vi "StellarNet MS Sw ini read I32.vi"(3 "Error State (In)":errorcluster, 4 "Section":string, 5 "configuration file path":path, 6 "Keys":string[](array[string])=["C1a", "C1b", "C1c", "C2d"]) -> (0 "Error State (Out)":errorcluster, 1 "Multi Elements":i32[](array[numeric]), 2 "Single Element":i32)   [LabVIEW 2023]
uses:
  <vilib>/Utility/config.llb/Read Key (I32).vi
  <vilib>/Utility/config.llb/NI_LVConfig.lvlib
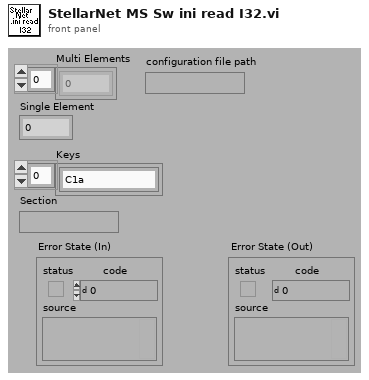
[diagram p1: front panel]
types:
  T1 = typedef "NI_LVConfig.lvlib/Config Data RefNum.ctl" = refnum<k1>
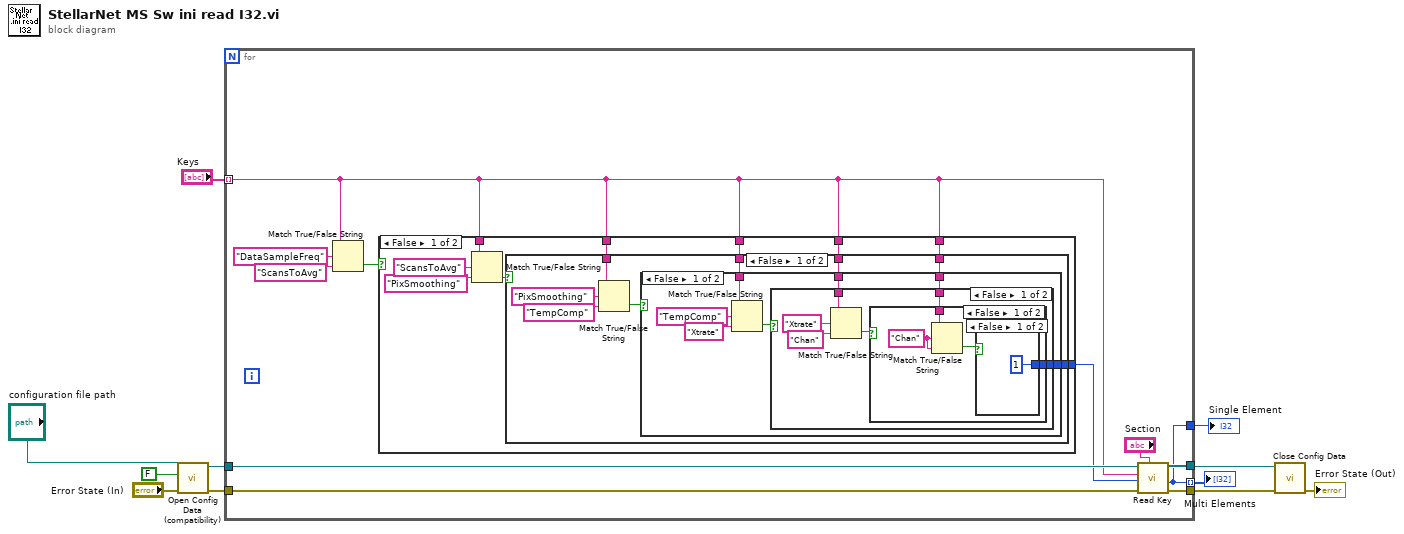
[diagram p0: block diagram]
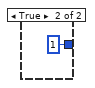
[diagram p2: hidden frame]
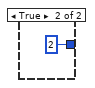
[diagram p3: hidden frame]
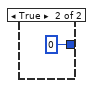
[diagram p4: hidden frame]
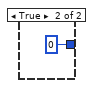
[diagram p5: hidden frame]
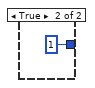
[diagram p6: hidden frame]
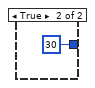
[diagram p7: hidden frame]
diagram:
  n1 = call <vilib>:"Open Config Data (compatibility).vi"("error in (no error)"="Error State (In)", "create file if necessary (T)"=FALSE ("create file if necessary? (T)"), "configuration file path"="configuration file path") -> ("error out"=w10:errorcluster, "refnum"=w9:T1)  [unwired: 6 in, 1 out]
  n2 = for {
    tunnel: w10 -> [w22]
    tunnel: w9 -> [w21]
    tunnel: "Keys" -> [w14] mode=indexing
    tunnel: [w18] -> w6 mode=indexing
    tunnel: [w20] -> w8
    tunnel: [w19] -> w7
    tunnel: [w18] -> w5
    n3 = Match True/False String(2:"ScansToAvg" ("regular expression"), 3:"DataSampleFreq" ("regular expression"), 4:w14) -> (0:w16:bool)  [unwired: 1 out]
    n4 = case shown="False" w16 {
      tunnel: w14 -> [w29 _]
      tunnel: w14 -> [w28 _]
      tunnel: w14 -> [w27 _]
      tunnel: w14 -> [w26 _]
      tunnel: w14 -> [w25 _]
      tunnel: [w24 30] -> w13
      frame False {
        n5 = Match True/False String(2:"PixSmoothing" ("regular expression"), 3:"ScansToAvg" ("regular expression"), 4:w29) -> (0:w30:bool)  [unwired: 1 out]
        n6 = case shown="False" w30 {
          tunnel: w28 -> [w38 _]
          tunnel: w27 -> [w36 _]
          tunnel: w26 -> [w35 _]
          tunnel: w25 -> [w34 _]
          tunnel: [w33 1] -> w24
          frame False {
            n7 = Match True/False String(2:"TempComp" ("regular expression"), 3:"PixSmoothing" ("regular expression"), 4:w38) -> (0:w37:bool)  [unwired: 1 out]
            n8 = case shown="False" w37 {
              tunnel: w36 -> [w45 _]
              tunnel: w35 -> [w44 _]
              tunnel: w34 -> [w42 _]
              tunnel: [w41 0] -> w33
              frame False {
                n9 = Match True/False String(2:"Xtrate" ("regular expression"), 3:"TempComp" ("regular expression"), 4:w45) -> (0:w43:bool)  [unwired: 1 out]
                n10 = case shown="False" w43 {
                  tunnel: w44 -> [w51 _]
                  tunnel: w42 -> [w49 _]
                  tunnel: [w48 0] -> w41
                  frame False {
                    n11 = Match True/False String(2:"Chan" ("regular expression"), 3:"Xtrate" ("regular expression"), 4:w51) -> (0:w50:bool)  [unwired: 1 out]
                    n12 = case shown="False" w50 {
                      tunnel: w49 -> [w56 _]
                      tunnel: [w54 2] -> w48
                      frame False {
                        w53 = "Chan" ("regular expression")
                        n13 = Match True/False String(2:w53, 3:w53, 4:w56) -> (0:w55:bool)  [unwired: 1 out]
                        n14 = case shown="False" w55 {
                          tunnel: [1 1] -> w54
                          frame False {
                          }
                          frame True {
                          }
                        }
                      }
                      frame True {
                      }
                    }
                  }
                  frame True {
                  }
                }
              }
              frame True {
              }
            }
          }
          frame True {
          }
        }
      }
      frame True {
      }
    }
    n15 = call-poly <vilib>:"Read Key.vi"("section"="Section", "error in (no error)"=w22, "default value"=w13, "key"=w14, "refnum"=w21) -> ("error out"=w19:errorcluster, "value"=w18:i32, "refnum out"=w20:T1)  [unwired: 3 in, 1 out]
  }
  "Multi Elements" <- w6
  "Single Element" <- w5
  n16 = call <vilib>:"Close Config Data.vi"("error in (no error)"=w7, "refnum"=w8) -> ("error out"=→"Error State (Out)":errorcluster)  [unwired: 8 in, 1 out]
